vi "Get Executable Version Information_LV2012_NI Verified.vi"(8 "error in (no error)":errorcluster) -> (0 "error out":errorcluster, 2 "FileVersion":string)   [LabVIEW 2012]
doc: "This VI returns the File Version of the Executable calling this function"
panel:
  # "Overview: This VI returns the File Version of the Executable calling this function\nRequirements: LabVIEW 2012 (or compatible), .NET Framework 3.5 (or Compatible)\nInstructions:\n1. Call this Function inside an exe application \n2. Launch the Executable"
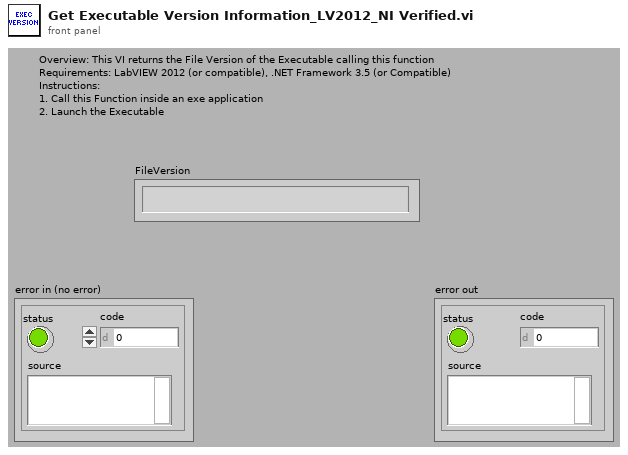
[diagram p1: front panel]
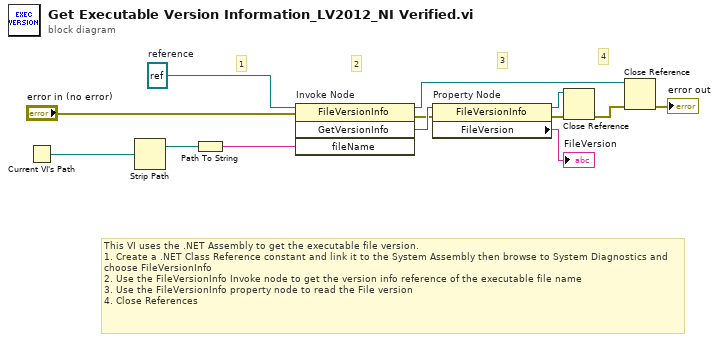
[diagram p0: block diagram]
diagram:
  w13 = refnum<k24> refnum  # reference
  # "4"
  # "3"
  # "2"
  # "1"
  # "This VI uses the .NET Assembly to get the executable file version.\n1. Create a .NET Class Reference constant and link it to the System Assembly then browse to System Diagnostics and choose FileVersionInfo\n2. Use the FileVersionInfo Invoke node to get the version info reference of the executable file name\n3. Use the FileVersionInfo property node to read the File version\n4. Close References"
  n1 = Current VI's Path() -> (path=w12:path)
  n2 = Strip Path(path=w12) -> (stripped path=w11:path)  [unwired: 1 out]
  n3 = Path To String(path=w11) -> (string=w10:string)
  n4 = invoke on="Invoke Node" class="FileVersionInfo" method="GetVersionInfo"(reference=w13, error in="error in (no error)", "fileName"=w10) -> (reference out=w3:refnum<k24>, error out=w8:errorcluster, "GetVersionInfo"=w9:refnum<k24>)  [unwired: 1 in, 1 out]
  n5 = property on="Property Node" class="FileVersionInfo"(reference=w9, error in=w8) -> (reference out=w6:refnum<k24>, error out=w5:errorcluster, "FileVersion"=→"FileVersion":string)
  n6 = Close Reference(reference=w6, error in (no error)=w5) -> (error out=w4:errorcluster)
  n7 = Close Reference(reference=w3, error in (no error)=w4) -> (error out=→"error out":errorcluster)
